vi "lvHistoricalQuery.vi"(0 "Path to Python.exe":path=path "C:/ProgramData/Anaconda3/python.exe", 2 "startTime":string, 3 "endTime":string, 5 "error in (no error)":errorcluster, 7 "gaugeselection":bool[](array[boolean]), 8 "Path":path, 9 "SaveData":bool, 11 "tcselection":bool[](array[boolean]), 13 "expected":bool[](array[boolean])) -> (14 "Raw Python String Output":string, 19 "error out":errorcluster)   [LabVIEW 2017]
panel:
  out "Standard Error":string
  out "Return Code":i32
  # "1. Inputs - Set before running VI"
  # "2. Outputs"
  # "3. Errors - Both Standard and LabVIEW"
  # "A + B ="
  # "This VI sends inputs to a simple Python script, and returns its output.\n\nSee block diagram for code and comments"
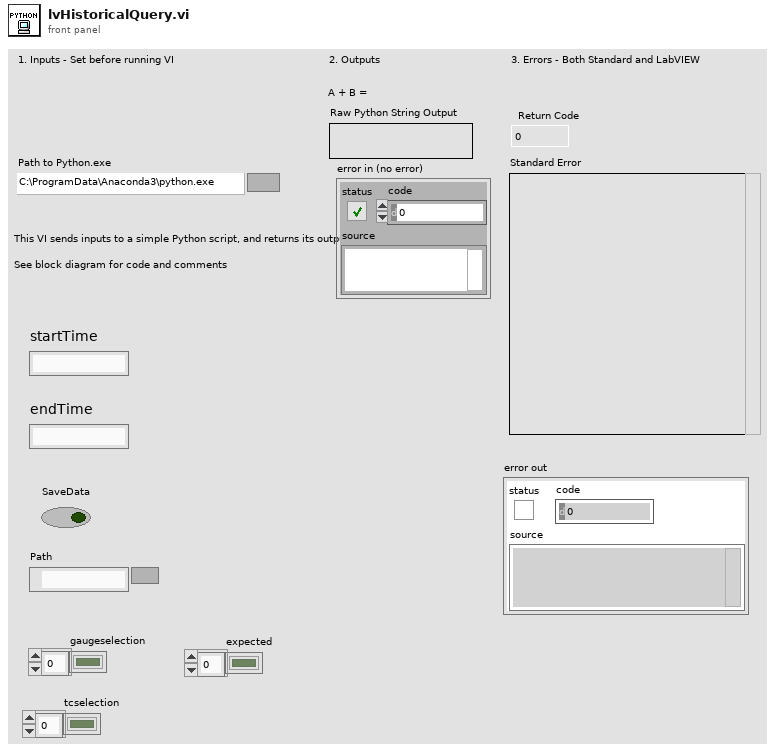
[diagram p1: front panel]
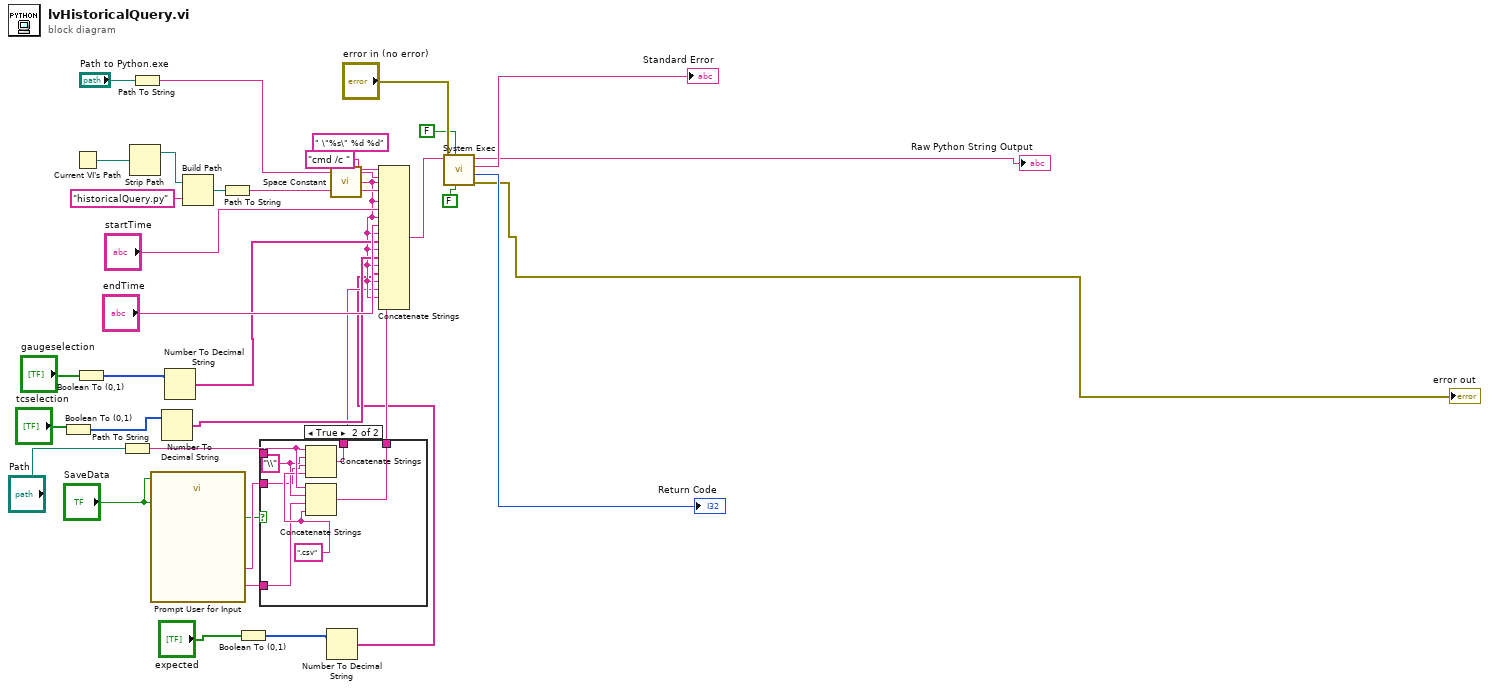
[diagram p0: block diagram]
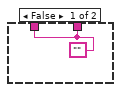
[diagram p2: hidden frame]
diagram:
  (unwired) " \"%s\" %d %d" ("format string")
  n1 = Boolean To (0,1)(Boolean="tcselection") -> (0, 1=w9:i16[])
  n2 = Current VI's Path() -> (path=w30:path)
  n3 = Boolean To (0,1)(Boolean="gaugeselection") -> (0, 1=w10:i16[])
  n4 = Path To String(path="Path") -> (string=w17:string)
  n5 = Strip Path(path=w30) -> (stripped path=w28:path)  [unwired: 1 out]
  n6 = Path To String(path="Path to Python.exe") -> (string=w25:string)
  n7 = call "Prompt User for Input"("Enable"="SaveData") -> ("Filename for Pressure"=w14:string, "Filename for Temperatures"=w15:string)  [unwired: 15 in, 2 out]
  n8 = Number To Decimal String(number=w9) -> (decimal integer string=w7:string[])  [unwired: 1 in]
  n9 = Number To Decimal String(number=w10) -> (decimal integer string=w8:string[])  [unwired: 1 in]
  n10 = Build Path(base path=w28, name or relative path="historicalQuery.py" ("Path to Function")) -> (appended path=w31:path)
  n11 = Path To String(path=w31) -> (string=w26:string)
  n12 = Boolean To (0,1)(Boolean="expected") -> (0, 1=w3:i16[])
  n13 = case shown="True" "SaveData" {
    tunnel: [w36 w43] -> w4
    tunnel: w17 -> [_ w42]
    tunnel: [w36 w41] -> w5
    tunnel: w15 -> [_ w38]
    tunnel: w14 -> [_ w37]
    frame False {
      w36 = ""
    }
    frame True {
      w40 = ".csv"
      w39 = "\\"
      n14 = Concatenate Strings(w42, w39, w38, w40) -> (w43:string)
      n15 = Concatenate Strings(w42, w39, w37, w40) -> (w41:string)
    }
  }
  n16 = Number To Decimal String(number=w3) -> (decimal integer string=w1:string[])  [unwired: 1 in]
  n17 = call <vilib>:"Space Constant.vi"() -> ("String"=w6:string)
  n18 = Concatenate Strings("cmd /c " ("string"), w25, w6, w26, w6, "startTime", w6, "endTime", w6, w8, w6, w7, w6, w1, w6, w4, w6, w5) -> (w27:string)
  n19 = call <vilib>:"System Exec.vi"("run minimized? (F)"=FALSE, "wait until completion? (T)"=FALSE, "error in (no error)"="error in (no error)", "command line"=w27) -> ("error out"=→"error out":errorcluster, "return code"=→"Return Code":i32, "standard error"=→"Standard Error":string, "standard output"=→"Raw Python String Output":string)  [unwired: 4 in]
